vi "USB - Asynchronous Write.vi"(8 "error in":errorcluster, 10 "Message to Send":string, 11 "VISA resource name in":refnum<visa-resource-name>) -> (0 "error out":errorcluster, 3 "VISA resource name out":refnum<visa-resource-name>)   [LabVIEW 2021]
doc: "Send an asynchronous message through USB/Serial"
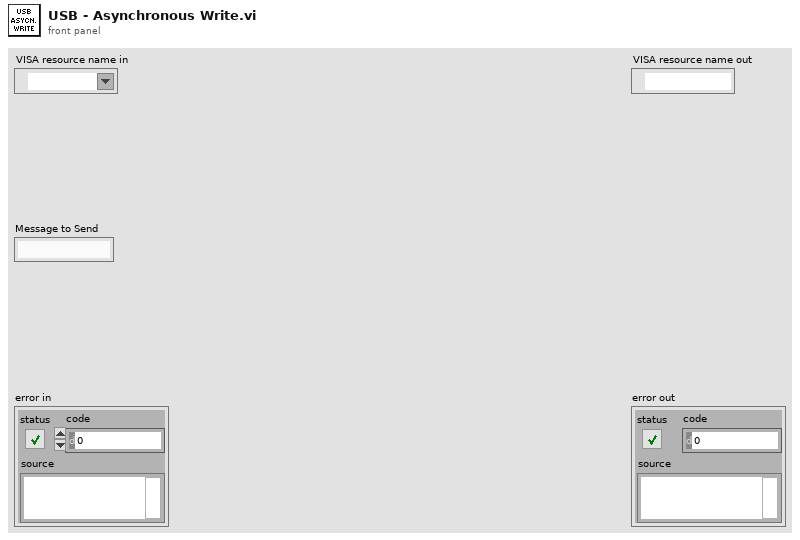
[diagram p1: front panel]
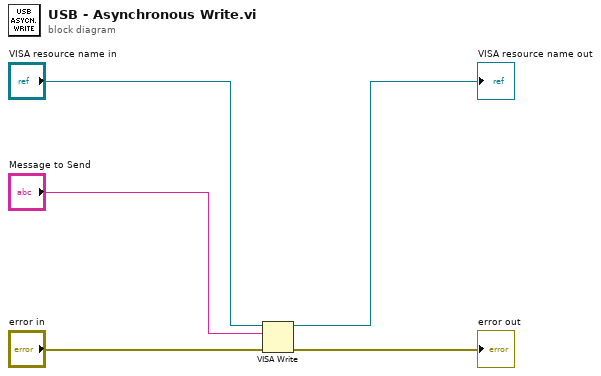
[diagram p0: block diagram]
diagram:
  n1 = VISA Write(VISA resource name="VISA resource name in", write buffer="Message to Send", error in (no error)="error in") -> (VISA resource name out=→"VISA resource name out":refnum<visa-resource-name>, error out=→"error out":errorcluster)  [unwired: 1 out]
